vi "Resample Blend.vi"(6 "Length":dbl=1.0, 8 "Speeds in":T1={"maxV (fps)"=20.0, "Accel Limit (fps^2)"=20.0, "Initial V (fps)"=0.0, "Sample Period (s)"=0.02, "Jerk Limit (fps^3)"=0.0, "Distances"=[]}, 9 "Initial Point":cluster{"x":dbl, "y":dbl, "th":dbl}={"x"=1.0, "y"=2.0, "th"=30.0}, 10 "Point Arrays":cluster{dbl[], dbl[], dbl[]}, 11 "Initial Acceleration":dbl format="%#_13g") -> (0 "Speeds out":T1={"maxV (fps)"=20.0, "Accel Limit (fps^2)"=20.0, "Initial V (fps)"=0.0, "Sample Period (s)"=0.02, "Jerk Limit (fps^3)"=0.0, "Distances"=[]}, 1 "Vel Points":cluster{dbl, dbl}[](array[cluster]), 2 "Points":cluster{dbl, dbl}[](array[cluster]), 3 "Indices":cluster{"Accel Index":i32, "Decel Index":i32}, 5 "Final Acceleration":dbl)   [LabVIEW 2019]
uses:
  Speeds.ctl
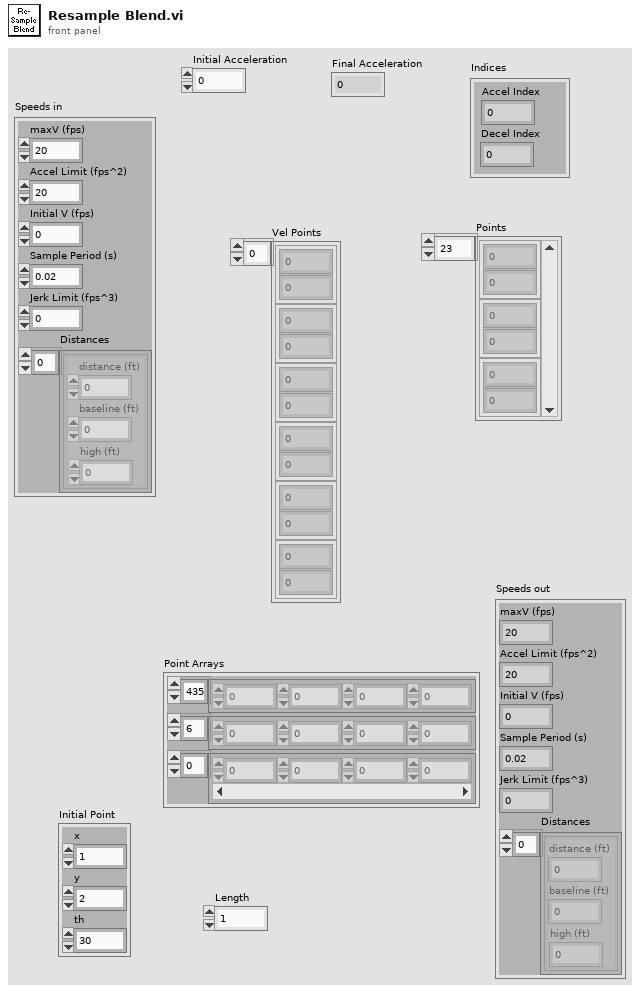
[diagram p1: front panel]
types:
  T1 = typedef "Speeds.ctl" = cluster{"maxV (fps)":dbl, "Accel Limit (fps^2)":dbl, "Initial V (fps)":dbl, "Sample Period (s)":dbl, "Jerk Limit (fps^3)":dbl, "Distances":cluster{"distance (ft)":dbl, "baseline (ft)":dbl, "high (ft)":dbl}[]}
  T2 = cluster{"distance (ft)":dbl, "baseline (ft)":dbl, "high (ft)":dbl}[]
  T3 = cluster{"Initial Acceleration":dbl, "Initial V (fps)":dbl}
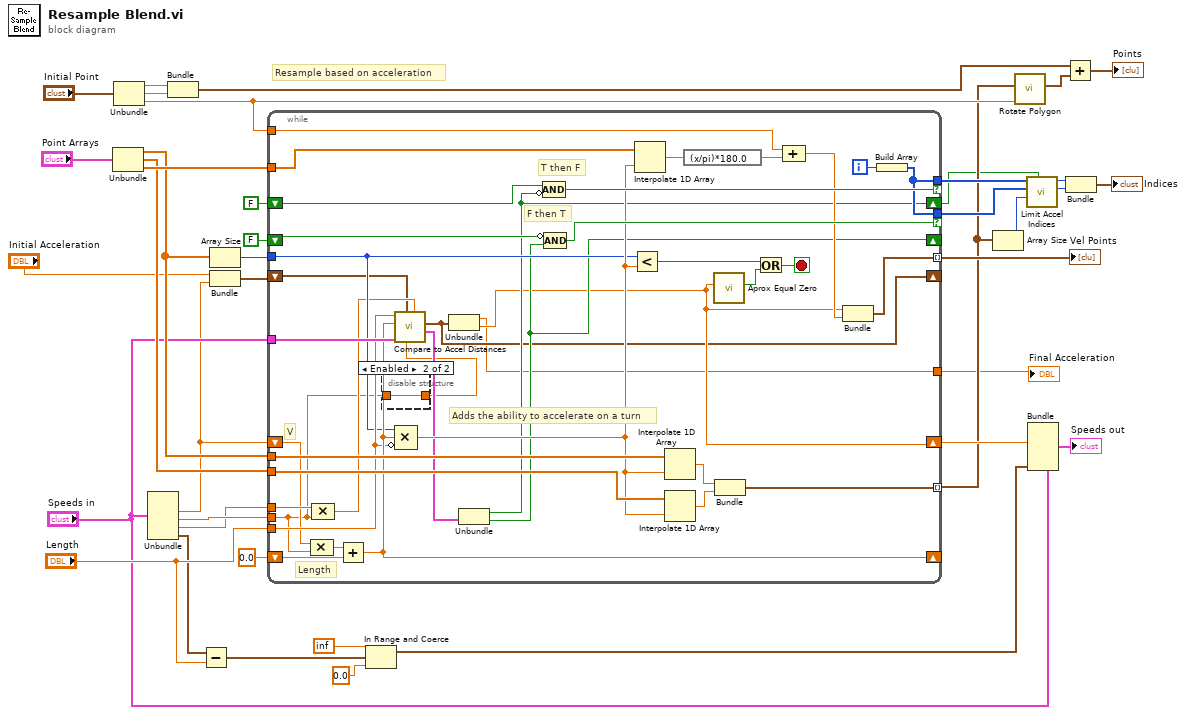
[diagram p0: block diagram]
diagram:
  # "Resample based on acceleration"
  n1 = Unbundle("Point Arrays") -> (w33:dbl[], w34:dbl[], w35:dbl[])
  n2 = Unbundle("Initial Point") -> ("x"=w30:dbl, "y"=w31:dbl, "th"=w29:dbl)
  n3 = Unbundle("Speeds in") -> ("Initial V (fps)"=w5:dbl, "Sample Period (s)"=w39:dbl, "Jerk Limit (fps^3)"=w8:dbl, "Distances"=w2:T2)  [unwired: 2 out]
  n4 = Bundle("x"=w30, "y"=w31) -> (w28:cluster{"x":dbl, "y":dbl})  [unwired: 1 in]
  n5 = Subtract(x=w2, y="Length") -> (x-y=w24:T2)
  n6 = Array Size(array=w33) -> (size(s)=w22:i32)
  n7 = Bundle("Initial Acceleration"="Initial Acceleration", "Initial V (fps)"=w5) -> (w7:T3)  [unwired: 1 in]
  n8 = while {
    tunnel: w33 -> [w78]
    tunnel: w34 -> [w77]
    tunnel: [w74] -> w15 mode=indexing
    tunnel: w39 -> [w41]
    shift-right: [w45] -> w38
    shift-left: w5 -> [w47]
    tunnel: w8 -> [w73]
    tunnel: w22 -> [w52]
    tunnel: w35 -> [w72]
    tunnel: w29 -> [w70]
    shift-right: [w49] -> w3
    shift-left: FALSE -> [w68]
    tunnel: [w56] -> w19 if=w67
    tunnel: "Length" -> [w54]
    tunnel: "Speeds in" -> [w66]
    shift-right: [w48] -> _
    shift-left: FALSE -> [w65]
    tunnel: [w56] -> w18 if=w64
    tunnel: [w61] -> w20 mode=indexing
    shift-right: [w55] -> _
    shift-left: 0.0 -> [w59]
    shift-right: [w44] -> _
    shift-left: w7 -> [w43]
    tunnel: [w40] -> w4
    i -> [w57]
    stop <- w62 stop-if-true
    # "F then T"
    # "T then F"
    # "Adds the ability to accelerate on a turn"
    # "Length"
    # "V"
    n9 = Compound Arithmetic op=MULTIPLY(w47, w41) -> (w58:dbl)
    n10 = Compound Arithmetic op=MULTIPLY(w73, w41) -> (w46:dbl)
    n11 = Add(x=w58, y=w59) -> (x+y=w55:dbl)
    n12 = disable-structure shown="Enabled" {
      disable-tunnel: [_ w79] -> w42
      disable-tunnel: w41 -> [_ w79]
      frame Disabled {
      }
      frame Enabled {
      }
    }
    n13 = call "Compare to Accel Distances.vi"("dA"=w46, "Sample Period (s)"=w42, "Values"=w43, "Speeds in"=w66, "Current  Length"=w55, "Total Segment Length"=w54) -> ("Ends"=w50:cluster{"Accel End":bool, "Decel End":bool}, "Values out"=w44:cluster{"accel":dbl, "velocity":dbl})  [unwired: 2 in, 2 out]
    n14 = Compound Arithmetic op=MULTIPLY(w52, w55, invert w54) -> (w53:dbl)
    n15 = Unbundle(w44) -> ("accel"=w40:dbl, "velocity"=w45:dbl)
    n16 = Unbundle(w50) -> ("Accel End"=w49:bool, "Decel End"=w48:bool)
    n17 = Compound Arithmetic op=AND(w68, invert w49) -> (w67:bool)
    n18 = Compound Arithmetic op=AND(invert w65, w48) -> (w64:bool)
    n19 = Less?(x=w52, y=w53) -> (x < y?=w63:bool)
    n20 = Interpolate 1D Array(1:w53, 2:w72) -> (0:w71:dbl)
    n21 = Interpolate 1D Array(1:w53, 2:w78) -> (0:w76:dbl)
    n22 = Interpolate 1D Array(1:w53, 2:w77) -> (0:w75:dbl)
    n23 = expression code="(x/pi)*180.0" ("radians to degrees")(w71) -> (w69:dbl)
    n24 = call "Aprox Equal Zero.vi"("maxV (fps)"=w45) -> ("Boolean"=w51:bool)  [unwired: 10 in]
    n25 = Bundle(w76, w75) -> (w74:cluster{dbl, dbl})  [unwired: 1 in]
    n26 = Or(x=w63, y=w51) -> (x .or. y?=w62:bool)
    n27 = Compound Arithmetic op=ADD(w70, w69) -> (w60:dbl)
    n28 = Bundle("velocity"=w45, w60) -> (w61:cluster{"velocity":dbl, dbl})  [unwired: 1 in]
    n29 = Build Array(w57) -> (w56:i32[])
  }
  "Vel Points" <- w20
  "Final Acceleration" <- w4
  n30 = In Range and Coerce(upper limit=inf, x=w24, lower limit=0.0) -> (coerced(x)=w1:T2)  [unwired: 1 out]
  n31 = Array Size(array=w15) -> (size(s)=w14:i32)
  n32 = call "Rotate Polygon.vi"("Angle"=w29, "polygon 2"=w15) -> ("polygon"=w27:cluster{dbl, dbl}[])  [unwired: 9 in]
  n33 = call "Limit Accel Indices.vi"("Last Accel"=w3, "Size"=w14, "Decel"=w18, "Accel"=w19) -> ("Decel Index"=w16:i32, "Accel Index"=w17:i32)  [unwired: 6 in]
  n34 = Bundle(cluster="Speeds in", "Initial V (fps)"=w38, "Distances"=w1) -> (→"Speeds out":T1)  [unwired: 4 in]
  n35 = Add(x=w28, y=w27) -> (x+y=→"Points":cluster{dbl, dbl}[])
  n36 = Bundle("Accel Index"=w17, "Decel Index"=w16) -> (→"Indices":cluster{"Accel Index":i32, "Decel Index":i32})  [unwired: 1 in]
